vi "Read error details.vi"(8 "error in (no error)":errorcluster, 11 "Printer_ZEBRA in":refnum<class "Printer_ZEBRA.lvclass">) -> (0 "error out":errorcluster, 2 "error details":errorcluster, 3 "Printer_ZEBRA out":refnum<class "Printer_ZEBRA.lvclass">)   [LabVIEW 2021, in "Printer_ZEBRA.lvclass"]
uses:
  Printer_ZEBRA.lvclass
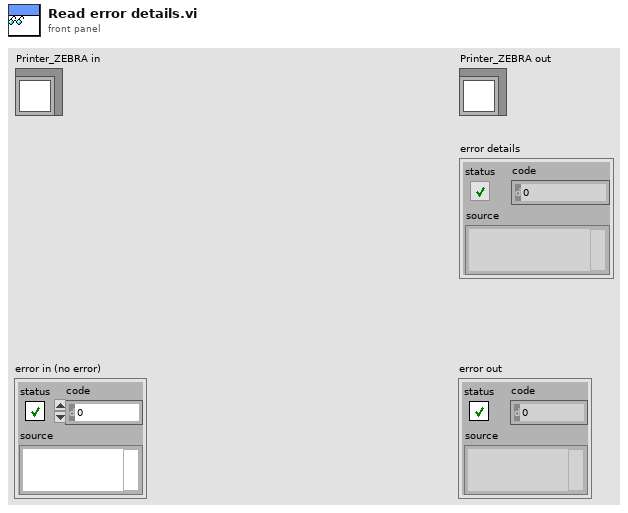
[diagram p1: front panel]
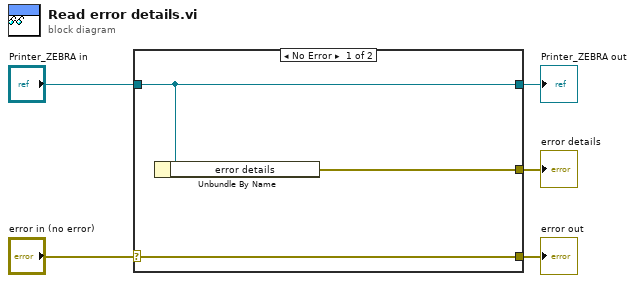
[diagram p0: block diagram]
diagram:
  n1 = case shown="No Error" "error in (no error)" {
    selector: "error in (no error)" -> [w8 w9]
    tunnel: [w8 w9] -> w4
    tunnel: [w7 w10] -> w2
    tunnel: "Printer_ZEBRA in" -> [w7 w10]
    tunnel: [w6 _] -> w1
    frame No Error {
      n2 = Unbundle By Name(w7) -> ("error details"=w6:errorcluster)
    }
    frame Error {
    }
  }
  "error out" <- w4
  "Printer_ZEBRA out" <- w2
  "error details" <- w1
